vi "RSZVB Get Marker Response.vi"(8 "error in (no error)":errorcluster {"code" format="%.0x"}, 9 "Marker (1)":i32=1, 10 "Channel (Trace) (1)":i32=1, 11 "VISA session":refnum<visa-resource-name>) -> (0 "error out":errorcluster {"code" format="%.0x"}, 2 "Marker Response":dbl[](array[numeric]) format="%^.3e", 3 "dup VISA session":refnum<visa-resource-name>)   [LabVIEW 2011]
doc: "This VI returns the response (in Cartesian diagrams: y-axis) value of marker no. <Mk>. The marker must be created before using CALCulate<Ch/Tr>:MARKer<Mk>[:STATe] ON.\n\nRemote-control command(s):\nCALCulate<Ch/Tr>:MARKer<Mk>:Y?"
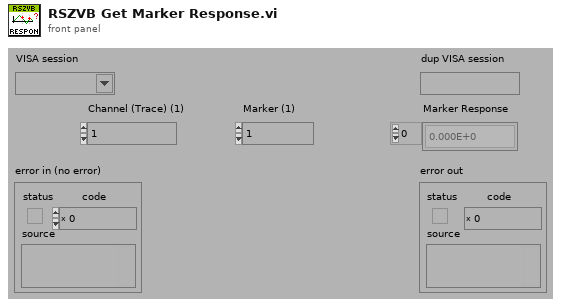
[diagram p1: front panel]
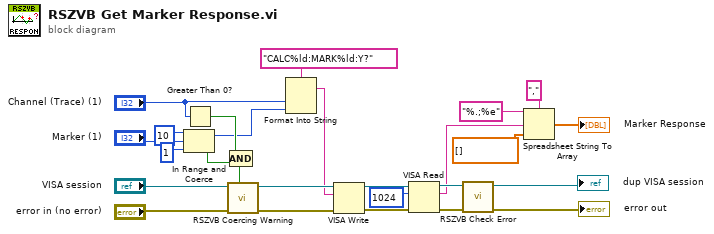
[diagram p0: block diagram]
diagram:
  n1 = In Range and Coerce(upper limit=10, x="Marker (1)", lower limit=1) -> (coerced(x)=w2:i32, In Range?=w15:bool)
  n2 = Greater Than 0?(x="Channel (Trace) (1)") -> (x > 0?=w14:bool)
  n3 = Compound Arithmetic op=AND(w14, w15) -> (w16:bool)
  n4 = call "RSZVB Coercing Warning.vi"("In Range?"=w16, "error in (no error)"="error in (no error)", "VISA session"="VISA session") -> ("error out"=w24:errorcluster, "dup VISA session"=w25:refnum<visa-resource-name>)  [unwired: 7 in]
  n5 = Format Into String(format string="CALC%ld:MARK%ld:Y?", "Channel (Trace) (1)", w2) -> (resulting string=w23:string)  [unwired: 2 in, 1 out]
  n6 = VISA Write(VISA resource name=w25, write buffer=w23, error in (no error)=w24) -> (VISA resource name out=w17:refnum<visa-resource-name>, error out=w18:errorcluster)  [unwired: 1 out]
  n7 = VISA Read(VISA resource name=w17, byte count=u32 1024 ("byte count (0)"), error in (no error)=w18) -> (VISA resource name out=w21:refnum<visa-resource-name>, read buffer=w13:string, error out=w20:errorcluster)  [unwired: 1 out]
  n8 = call "RSZVB Check Error.vi"("error in (no error)"=w20, "VISA session"=w21) -> ("error out"=→"error out":errorcluster, "dup VISA session"=→"dup VISA session":refnum<visa-resource-name>)  [unwired: 8 in]
  n9 = Spreadsheet String To Array(delimiter (Tab)=",", format string="%.;%e", spreadsheet string=w13, array type (2D Dbl)=dbl[] []) -> (array=→"Marker Response":dbl[])
